vi "UTS - Expected Response Trigger.vi"(9 "String Buffer in":string, 11 "Expected Response":T1) -> (1 "String Buffer out":string, 2 "Expected Response triggered":bool, 3 "Response":string)   [LabVIEW 2017, in "SSH.lvlib"]
uses:
  SSH.lvlib
  Expected Response String Config.ctl
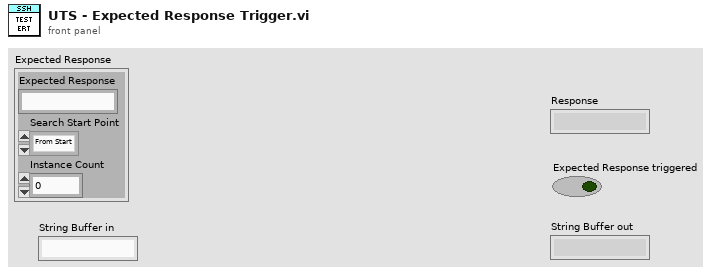
[diagram p1: front panel]
types:
  T1 = typedef "SSH.lvlib/Expected Response String Config.ctl" = cluster{"Expected Response":string, "Search Start Point":enum16{"From Start", "From End"}, "Instance Count":i32}
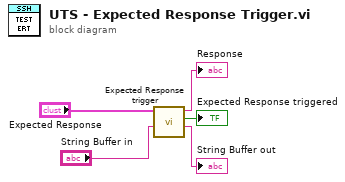
[diagram p0: block diagram]
diagram:
  n1 = call "Expected Response trigger.vi"("String Buffer in"="String Buffer in", "Expected Response"="Expected Response") -> ("String Buffer out"=→"String Buffer out":string, "Expected Response triggered"=→"Expected Response triggered":bool, "Response"=→"Response":string)  [unwired: 7 in]
